vi "ARM PROJECT.vi"() -> ()   [LabVIEW 2020]
panel:
  in  "RE-UP":bool
  in  "RE":bool
  in  "Down-R":bool
  in  "R-L":bool
  in  "Up":bool
  in  "Hold":bool
  in  "Down":bool
  out "Bottle":bool
  out "ARM":bool
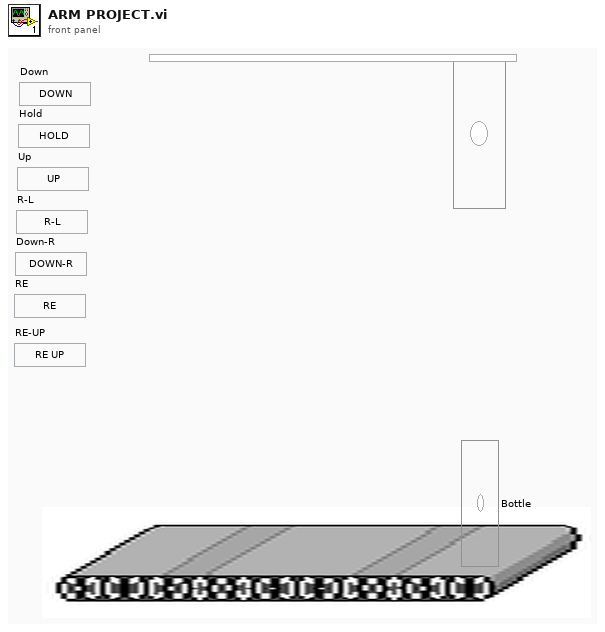
[diagram p1: front panel]
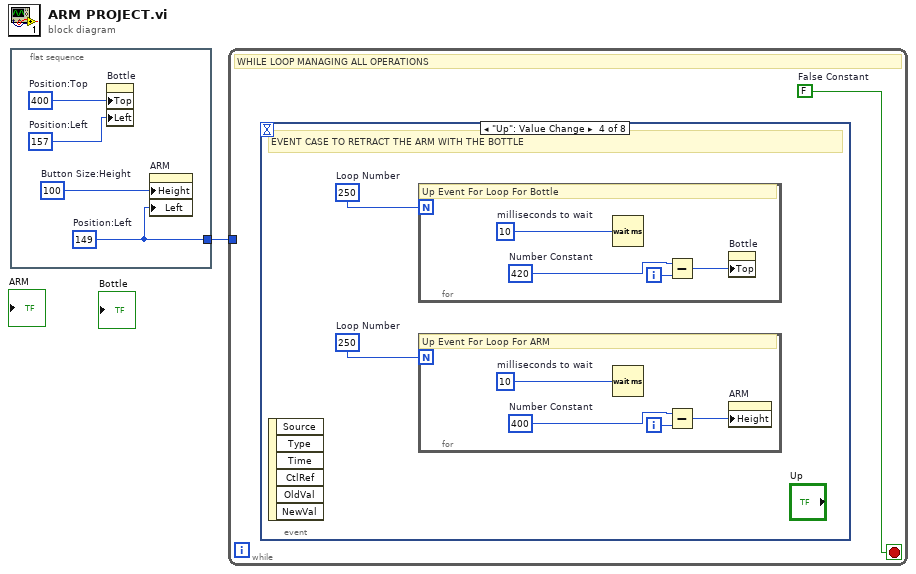
[diagram p0: block diagram]
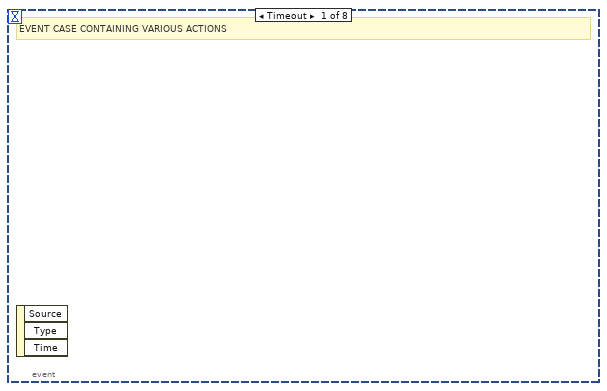
[diagram p2: hidden frame]
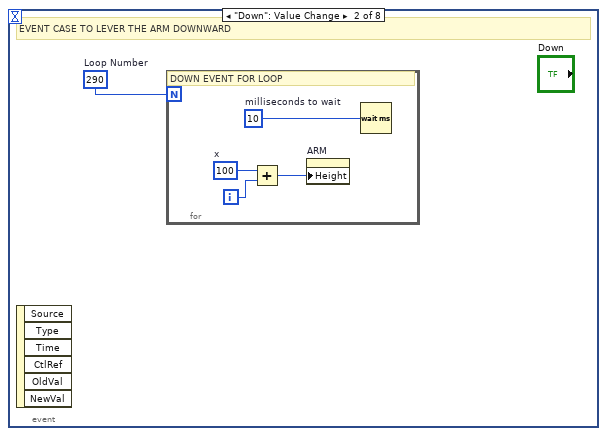
[diagram p3: hidden frame]
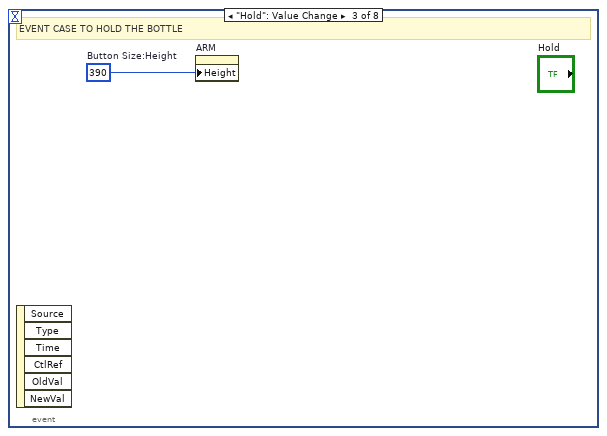
[diagram p4: hidden frame]
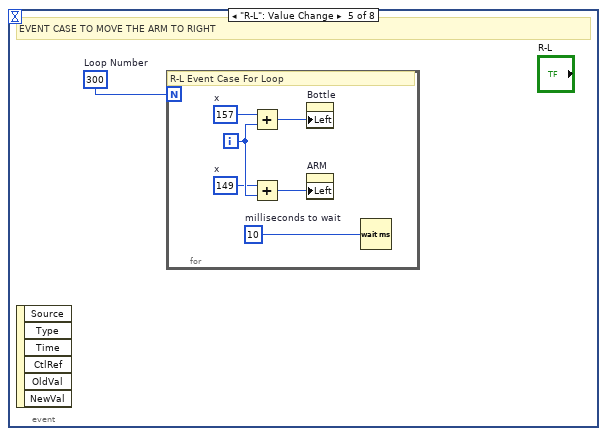
[diagram p5: hidden frame]
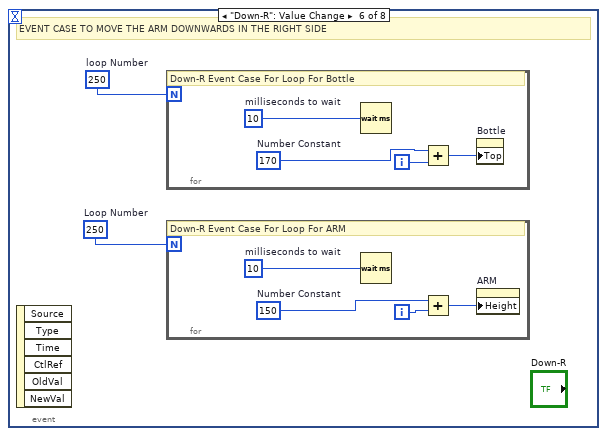
[diagram p6: hidden frame]
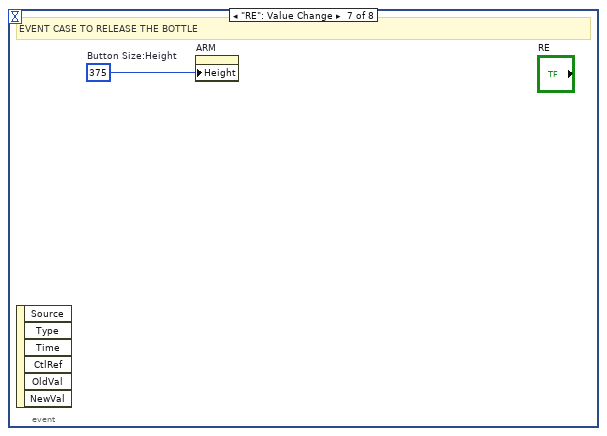
[diagram p7: hidden frame]
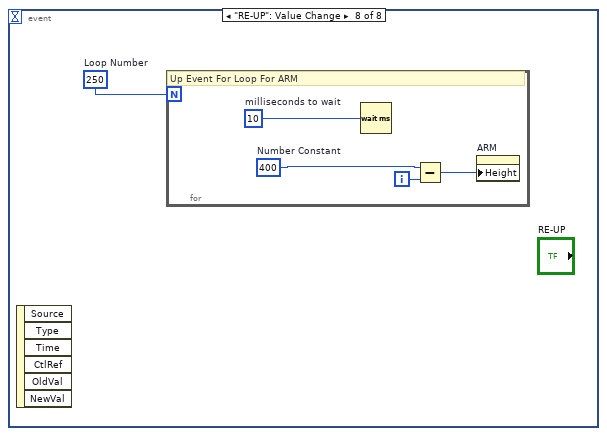
[diagram p8: hidden frame]
diagram:
  n1 = flat-sequence {
    tunnel: [w2] -> w1
    frame #0 {
      w3 = 157  # Position:Left
      w2 = 149  # Position:Left
      w4 = 400  # Position:Top
      w5 = u32 100  # Button Size:Height
      n2 = property on="Bottle" class="Bool (strict)"("Top"=w4, "Left"=w3) -> ()  [unwired: 2 in, 2 out]
      n3 = property on="ARM" class="Bool (strict)"("Height"=w5, "Left"=w2) -> ()  [unwired: 2 in, 2 out]
    }
  }
  n4 = while {
    tunnel: w1 -> [_]
    stop <- w6 stop-if-true
    w6 = FALSE  # False Constant
    # "WHILE LOOP MANAGING ALL OPERATIONS"
    n5 = event shown="[3] \"Up\": Value Change" {
      selector: _ -> [_ _ _ _ _ _ _ _]
      dyn-events: _ -> [_ _ _ _ _ _ _ _]
      timeout: _ -> [_ _ _ _ _ _ _ _]
      event Timeout {
        # "EVENT CASE CONTAINING VARIOUS ACTIONS"
        n6 = event-data() -> ()  [unwired: 1 in, 3 out]
      }
      event "Down": Value Change {
        w7 = 290  # Loop Number
        # "EVENT CASE TO LEVER THE ARM DOWNWARD"
        n7 = event-data() -> ()  [unwired: 1 in, 6 out]
        n8 = for {
          N: w7 -> [_]
          i -> [w8]
          w9 = 100  # x
          w11 = u32 10  # milliseconds to wait
          # "DOWN EVENT FOR LOOP"
          n9 = Add(x=w9, y=w8) -> (x+y=w10:i32)
          n10 = property on="ARM" class="Bool (strict)"("Height"=w10) -> ()  [unwired: 2 in, 2 out]
          n11 = Wait (ms)(milliseconds to wait=w11) -> ()  [unwired: 1 out]
        }
      }
      event "Hold": Value Change {
        w12 = u32 390  # Button Size:Height
        # "EVENT CASE TO HOLD THE BOTTLE"
        n12 = event-data() -> ()  [unwired: 1 in, 6 out]
        n13 = property on="ARM" class="Bool (strict)"("Height"=w12) -> ()  [unwired: 2 in, 2 out]
      }
      event "Up": Value Change {
        w13 = 250  # Loop Number
        w14 = 250  # Loop Number
        # "EVENT CASE TO RETRACT THE ARM WITH THE BOTTLE"
        n14 = event-data() -> ()  [unwired: 1 in, 6 out]
        n15 = for {
          N: w14 -> [_]
          i -> [w20]
          w19 = u32 10  # milliseconds to wait
          w21 = 420  # Number Constant
          # "Up Event For Loop For Bottle"
          n16 = Wait (ms)(milliseconds to wait=w19) -> ()  [unwired: 1 out]
          n17 = Subtract(x=w21, y=w20) -> (x-y=w22:i32)
          n18 = property on="Bottle" class="Bool (strict)"("Top"=w22) -> ()  [unwired: 2 in, 2 out]
        }
        n19 = for {
          N: w13 -> [_]
          i -> [w16]
          w15 = u32 10  # milliseconds to wait
          w18 = 400  # Number Constant
          # "Up Event For Loop For ARM"
          n20 = Wait (ms)(milliseconds to wait=w15) -> ()  [unwired: 1 out]
          n21 = Subtract(x=w18, y=w16) -> (x-y=w17:i32)
          n22 = property on="ARM" class="Bool (strict)"("Height"=w17) -> ()  [unwired: 2 in, 2 out]
        }
      }
      event "R-L": Value Change {
        w23 = 300  # Loop Number
        # "EVENT CASE TO MOVE THE ARM TO RIGHT"
        n23 = event-data() -> ()  [unwired: 1 in, 6 out]
        n24 = for {
          N: w23 -> [_]
          i -> [w27]
          w24 = u32 10  # milliseconds to wait
          w25 = 157  # x
          w26 = 149  # x
          # "R-L Event Case For Loop"
          n25 = Add(x=w25, y=w27) -> (x+y=w29:i32)
          n26 = Add(x=w26, y=w27) -> (x+y=w28:i32)
          n27 = property on="Bottle" class="Bool (strict)"("Left"=w29) -> ()  [unwired: 2 in, 2 out]
          n28 = property on="ARM" class="Bool (strict)"("Left"=w28) -> ()  [unwired: 2 in, 2 out]
          n29 = Wait (ms)(milliseconds to wait=w24) -> ()  [unwired: 1 out]
        }
      }
      event "Down-R": Value Change {
        w30 = 250  # Loop Number
        w31 = 250  # loop Number
        # "EVENT CASE TO MOVE THE ARM DOWNWARDS IN THE RIGHT SIDE"
        n30 = event-data() -> ()  [unwired: 1 in, 6 out]
        n31 = for {
          N: w31 -> [_]
          i -> [w33]
          w32 = u32 10  # milliseconds to wait
          w34 = 170  # Number Constant
          # "Down-R Event Case For Loop For Bottle"
          n32 = Wait (ms)(milliseconds to wait=w32) -> ()  [unwired: 1 out]
          n33 = Add(x=w34, y=w33) -> (x+y=w35:i32)
          n34 = property on="Bottle" class="Bool (strict)"("Top"=w35) -> ()  [unwired: 2 in, 2 out]
        }
        n35 = for {
          N: w30 -> [_]
          i -> [w37]
          w36 = u32 10  # milliseconds to wait
          w39 = 150  # Number Constant
          # "Down-R Event Case For Loop For ARM"
          n36 = Wait (ms)(milliseconds to wait=w36) -> ()  [unwired: 1 out]
          n37 = Add(x=w39, y=w37) -> (x+y=w38:i32)
          n38 = property on="ARM" class="Bool (strict)"("Height"=w38) -> ()  [unwired: 2 in, 2 out]
        }
      }
      event "RE": Value Change {
        w40 = u32 375  # Button Size:Height
        # "EVENT CASE TO RELEASE THE BOTTLE"
        n39 = event-data() -> ()  [unwired: 1 in, 6 out]
        n40 = property on="ARM" class="Bool (strict)"("Height"=w40) -> ()  [unwired: 2 in, 2 out]
      }
      event "RE-UP": Value Change {
        w41 = 250  # Loop Number
        n41 = event-data() -> ()  [unwired: 1 in, 6 out]
        n42 = for {
          N: w41 -> [_]
          i -> [w43]
          w42 = u32 10  # milliseconds to wait
          w45 = 400  # Number Constant
          # "Up Event For Loop For ARM"
          n43 = Wait (ms)(milliseconds to wait=w42) -> ()  [unwired: 1 out]
          n44 = Subtract(x=w45, y=w43) -> (x-y=w44:i32)
          n45 = property on="ARM" class="Bool (strict)"("Height"=w44) -> ()  [unwired: 2 in, 2 out]
        }
      }
    }
  }
